vi "RequestStatus.vi"(8 "error in (no error) 2":errorcluster, 10 "Data":i32, 11 "Beta in":refnum<class "MyBaseActor.lvclass">) -> (0 "error out 2":errorcluster, 2 "x*y":i32, 3 "Beta out":refnum<class "MyBaseActor.lvclass">)   [LabVIEW 2016, in "MyBaseActor.lvlib" / "MyBaseActor.lvclass"]
uses:
  MyBaseActor.lvclass
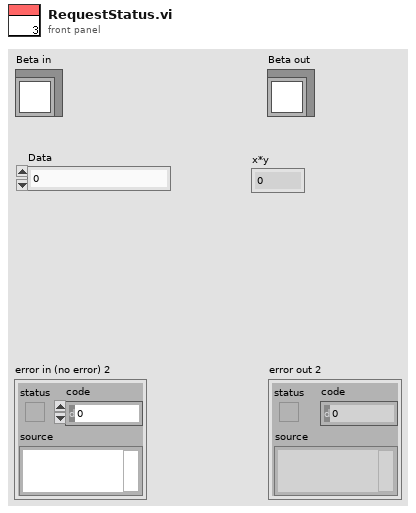
[diagram p1: front panel]
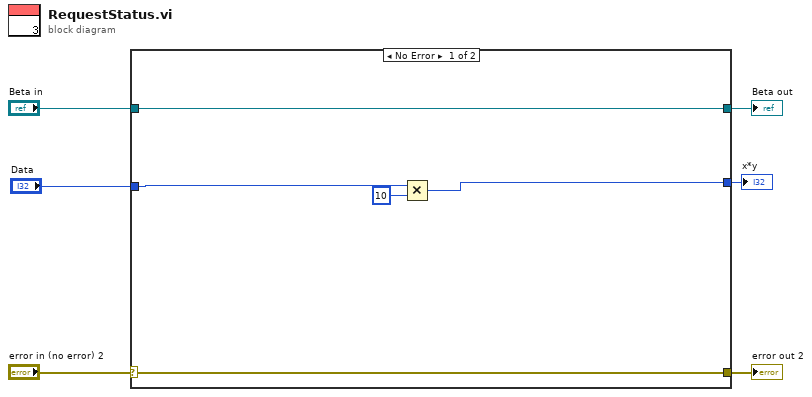
[diagram p0: block diagram]
diagram:
  n1 = case shown="No Error" "error in (no error) 2" {
    selector: "error in (no error) 2" -> [w11 w13]
    tunnel: [w11 w13] -> w5
    tunnel: [w10 w12] -> w3
    tunnel: "Beta in" -> [w10 w12]
    tunnel: "Data" -> [w9 _]
    tunnel: [w7 _] -> w1
    frame No Error {
      n2 = Multiply(x=w9, y=10) -> (x*y=w7:i32)
    }
    frame Error {
    }
  }
  "error out 2" <- w5
  "Beta out" <- w3
  "x*y" <- w1
